vi "SCE_enab_dis_row_col_screen.vi"(8 "row":i32, 9 "col":i32, 10 "char ID":i32, 11 "VIC-II":T1) -> (2 "char ID out":i32)   [LabVIEW 2018]
uses:
  SCE_VIC-II_registry.ctl
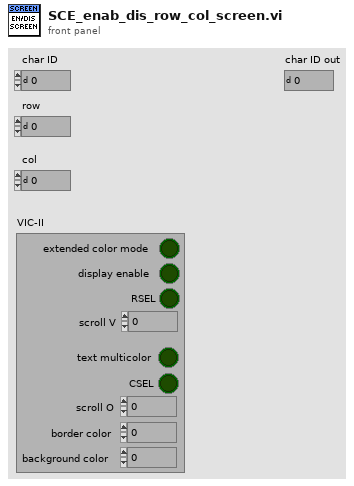
[diagram p1: front panel]
types:
  T1 = typedef "SCE_VIC-II_registry.ctl" = cluster{"extended color mode":bool, "display enable":bool, "RSEL":bool, "scroll V":u8, "text multicolor":bool, "CSEL":bool, "scroll O":u8, "border color":u8, "background color":u8}
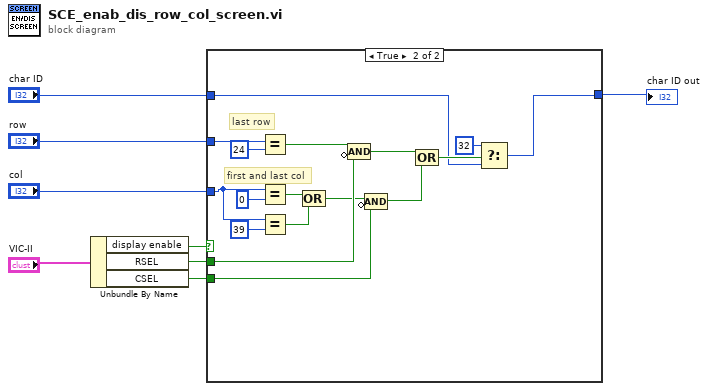
[diagram p0: block diagram]
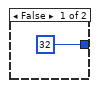
[diagram p2: hidden frame]
diagram:
  n1 = Unbundle By Name("VIC-II") -> ("display enable"=w7:bool, "RSEL"=w2:bool, "CSEL"=w1:bool)
  n2 = case shown="True" w7 {
    tunnel: "char ID" -> [_ w12]
    tunnel: "row" -> [_ w26]
    tunnel: "col" -> [_ w20]
    tunnel: [32 ("char ID out") w10] -> w3
    tunnel: w2 -> [_ w23]
    tunnel: w1 -> [_ w16]
    frame False {
    }
    frame True {
      # "first and last col"
      # "last row"
      n3 = Equal?(x=w26, y=24) -> (x = y?=w24:bool)
      n4 = Equal?(x=w20, y=0) -> (x = y?=w19:bool)
      n5 = Equal?(x=w20, y=39) -> (x = y?=w18:bool)
      n6 = Compound Arithmetic op=OR(w19, w18) -> (w17:bool)
      n7 = Compound Arithmetic op=AND(w24, invert w23) -> (w15:bool)
      n8 = Compound Arithmetic op=AND(w17, invert w16) -> (w14:bool)
      n9 = Compound Arithmetic op=OR(w15, w14) -> (w13:bool)
      n10 = Select(t=32, s=w13, f=w12) -> (s? t:f=w10:i32)
    }
  }
  "char ID out" <- w3
